vi "Event Handle Dispatcher.vi"(8 "error in (no error)":errorcluster, 11 "QMenu Class in":refnum<class "QMenu Class.lvclass">) -> (0 "error out":errorcluster)   [LabVIEW 2020, in "QTab.lvlib" / "QMenu Class.lvclass"]
uses:
  QMenu Class.lvclass
  Command.ctl
  QMenu Class.lvclass/QMenu Class.ctl
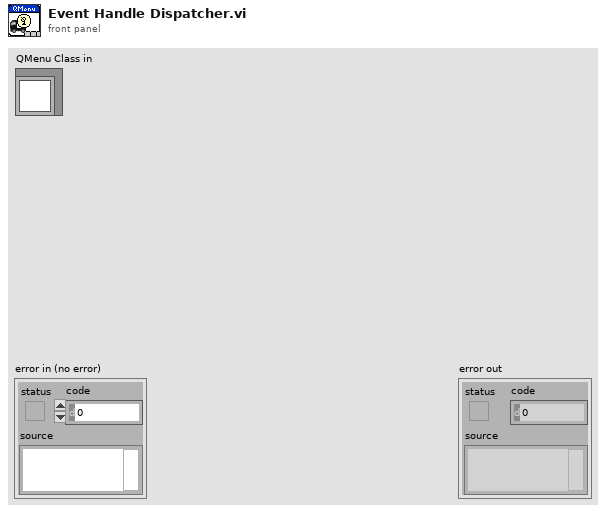
[diagram p1: front panel]
types:
  T1 = typedef "QTab.lvlib/QMenu Class.lvclass/Command.ctl" = enum16{"Initialize", "Get Active Button", "Set Active Button", "Set Button Attribute", "Add Button", "Close Button", "Draw", "Stop"}
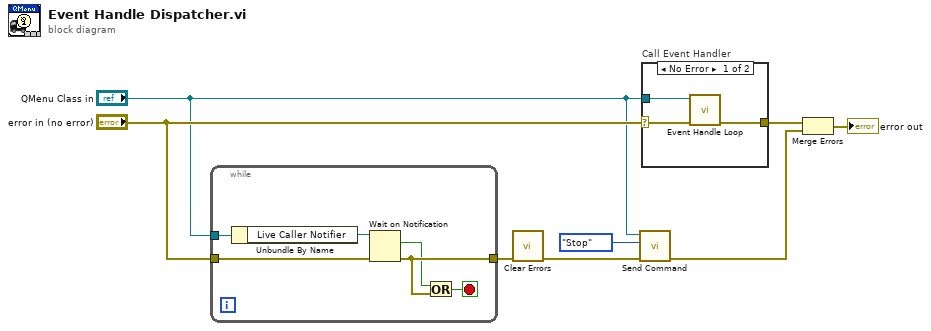
[diagram p0: block diagram]
diagram:
  n1 = while {
    tunnel: "QMenu Class in" -> [w12]
    tunnel: "error in (no error)" -> [w13]
    tunnel: [w11] -> w2
    stop <- w9 stop-if-true
    n2 = Unbundle By Name(w12) -> ("Live Caller Notifier"=w14:refnum<notifier>)
    n3 = Wait on Notification(notifier=w14, error in (no error)=w13) -> (notification=w10:bool, error out=w11:errorcluster)  [unwired: 2 in, 2 out]
    n4 = Or(x=w10, y=w11) -> (x .or. y?=w9:bool)
  }
  n5 = call <vilib>:"Clear Errors.vi"("error in (no error)"=w2) -> ("error out"=w1:errorcluster)  [unwired: 5 in, 1 out]
  n6 = call "Send Command.vi"("error in (no error)"=w1, "Command"=Command."Stop", "QMenu Class in"="QMenu Class in") -> ("error out"=w4:errorcluster)  [unwired: 7 in, 1 out]
  n7 = case "Call Event Handler" shown="No Error" "error in (no error)" {
    selector: "error in (no error)" -> [w15 w18]
    tunnel: [w17 w18] -> w8
    tunnel: "QMenu Class in" -> [w16 _]
    frame No Error {
      n8 = call "Event Handle Loop.vi"("error in (no error)"=w15, "QMenu Class in"=w16) -> ("error out"=w17:errorcluster)  [unwired: 8 in, 1 out]
    }
    frame Error {
    }
  }
  n9 = Merge Errors(w8, w4) -> (→"error out":errorcluster)
